vi "rszvl_core_global.vi"() -> ()   [LabVIEW 2014] (continued)
Callback"="", "Write Callback"="", "Range Callback"="", "Check Callback"="", "Rngtable Callback"="", "Coerce Callback"="", "User Callback"="", "Supported Models"="", "Instrument Options"="", "Repeated Capabilities"="", "Restricted Repeated Capabilities"="", "Help"="This attribute initiates an instrument reset.\n\nAvailable Repeated Capabilities:\nNone\n\nRemote-control command(s):\nSYSTem:PRESet", "Flags"={"OPC Wait"=FALSE, "Dont check status"=FALSE, "*WAI"=FALSE}, "Check Status Callback"=""}, {"Level"=2, "Descriptive Name"="System Version", "Class Only"=FALSE, "Data Type"=2, "Access"=0, "Identifier"="RSZVL_ATTR_SYST_VERSION", "Range Table"="", "Command"="SYST:VERS?", "Read Callback"="", "Write Callback"="", "Range Callback"="", "Check Callback"="", "Rngtable Callback"="", "Coerce Callback"="", "User Callback"="", "Supported Models"="", "Instrument Options"="", "Repeated Capabilities"="", "Restricted Repeated Capabilities"="", "Help"="This attribute queries the system version.\n\nAvailable Repeated Capabilities:\nNone\n\nRemote-control command(s):\nSYSTem:VERSion?", "Flags"={"OPC Wait"=FALSE, "Dont check status"=FALSE, "*WAI"=FALSE}, "Check Status Callback"=""}, {"Level"=2, "Descriptive Name"="Speaker Volume", "Class Only"=FALSE, "Data Type"=1, "Access"=2, "Identifier"="RSZVL_ATTR_SYST_SPEAKER", "Range Table"="rszvl_rngSpeakerVolume", "Command"="SYST:SPE:VOL", "Read Callback"="", "Write Callback"="", "Range Callback"="", "Check Callback"="", "Rngtable Callback"="", "Coerce Callback"="", "User Callback"="", "Supported Models"="", "Instrument Options"="", "Repeated Capabilities"="", "Restricted Repeated Capabilities"="", "Help"="This attribute sets the volume of the built-in loudspeaker for demodulated signals.\n\nAvailable Repeated Capabilities:\nNone\n\nRemote-control command(s):\nSYSTem:SPEaker:VOLume", "Flags"={"OPC Wait"=FALSE, "Dont check status"=FALSE, "*WAI"=FALSE}, "Check Status Callback"=""}, {"Level"=1, "Descriptive Name"="NWA Channel", "Class Only"=TRUE, "Data Type"=0, "Access"=0, "Identifier"="", "Range Table"="", "Command"="", "Read Callback"="", "Write Callback"="", "Range Callback"="", "Check Callback"="", "Rngtable Callback"="", "Coerce Callback"="", "User Callback"="", "Supported Models"="", "Instrument Options"="", "Repeated Capabilities"="", "Restricted Repeated Capabilities"="", "Help"="(1) NWA Number Of Sweeps:\nThis attribute defines the number of sweeps to be measured in single sweep mode (INITiate<Ch>:CONTinuous OFF). \n\n(2) NWA Averaging State:\nThis attribute enable or disable the sweep average.\n\n(3) NWA Averaging Count:\nThis attribute defines the number of consecutive sweeps to be combined for the sweep average (Average Factor).\n\n(4) NWA Restart Average:\nThis attribute starts a new average cycle, clearing all previous results and thus eliminating their effect on the new cycle. \n\n(5) NWA Resolution Bandwidth:\nThis attribute defines the resolution bandwidth of the analyzer (Meas Bandwidth).\n\n(6) NWA Sweep Points:\nThis attribute defines the total number of measurement points per sweep (Number of Points).\n\n(7) NWA Channel State:\nThis attribute creates or deletes channel no. <Ch> and selects it as the active channel. \n\n(8) NWA Channel Name:\nThis attribute assigns a name to channel number <Ch>. The channel must be created before (CONFigure:CHANnel<Ch>[:STATe] ON). Moreover it is not possible to assign the same name to two different channels.\n\n(9) NWA Assign Trace:\nThis attribute assigns an existing trace to a diagram area, using the <WndTr> suffix, and displays the trace.", "Flags"={"OPC Wait"=FALSE, "Dont check status"=FALSE, "*WAI"=FALSE}, "Check Status Callback"=""}, {"Level"=2, "Descriptive Name"="NWA Number Of Sweeps", "Class Only"=FALSE, "Data Type"=0, "Access"=2, "Identifier"="RSZVL_ATTR_NWA_NUMBER_OF_SWEEPS", "Range Table"="rszvl_rngNWANumberOfSweeps", "Command"="SENS:SWE:COUN", "Read Callback"="", "Write Callback"="", "Range Callback"="", "Check Callback"="", "Rngtable Callback"="", "Coerce Callback"="", "User Callback"="", "Supported Models"="", "Instrument Options"="", "Repeated Capabilities"="", "Restricted Repeated Capabilities"="", "Help"="This attribute defines the number of sweeps to be measured in single sweep mode (INITiate<Ch>:CONTinuous OFF).\n\nAvailable Repeated Capabilities:\nNone\n\nRemote-control command(s):\n[SENSe<1|2>:]SWEep:COUNt", "Flags"={"OPC Wait"=FALSE, "Dont check status"=FALSE, "*WAI"=FALSE}, "Check Status Callback"=""}, {"Level"=2, "Descriptive Name"="NWA Averaging State", "Class Only"=FALSE, "Data Type"=3, "Access"=2, "Identifier"="RSZVL_ATTR_NWA_AVG_STATE", "Range Table"="", "Command"="SENS{Channel}:AVER:STAT", "Read Callback"="", "Write Callback"="", "Range Callback"="", "Check Callback"="", "Rngtable Callback"="", "Coerce Callback"="", "User Callback"="", "Supported Models"="", "Instrument Options"="", "Repeated Capabilities"="", "Restricted Repeated Capabilities"="", "Help"="This attribute enable or disable the sweep average.\n\nAvailable Repeated Capabilities:\nChannel: CH1,CH2,CH3,CH4,CH5,CH6,CH7,CH8,CH9,CH10,CH11,CH12,CH13,CH14,CH15,CH16,CH17,CH18,CH19,CH20\r\n\nRemote-control command(s):\n[SENSe<Ch>:]AVERage[:STATe] ON | OFF", "Flags"={"OPC Wait"=FALSE, "Dont check status"=FALSE, "*WAI"=FALSE}, "Check Status Callback"=""}, {"Level"=2, "Descriptive Name"="NWA Averaging Count", "Class Only"=FALSE, "Data Type"=0, "Access"=2, "Identifier"="RSZVL_ATTR_NWA_AVG_COUNT", "Range Table"="rszvl_rngNWAAvgCount", "Command"="SENS{Channel}:AVER:COUN", "Read Callback"="", "Write Callback"="", "Range Callback"="", "Check Callback"="", "Rngtable Callback"="", "Coerce Callback"="", "User Callback"="", "Supported Models"="", "Instrument Options"="", "Repeated Capabilities"="", "Restricted Repeated Capabilities"="", "Help"="This attribute defines the number of consecutive sweeps to be combined for the sweep average (Average Factor).\n\nAvailable Repeated Capabilities:\nChannel: CH1,CH2,CH3,CH4,CH5,CH6,CH7,CH8,CH9,CH10,CH11,CH12,CH13,CH14,CH15,CH16,CH17,CH18,CH19,CH20\r\n\nRemote-control command(s):\n[SENSe<Ch>:]AVERage:COUNt", "Flags"={"OPC Wait"=FALSE, "Dont check status"=FALSE, "*WAI"=FALSE}, "Check Status Callback"=""}, {"Level"=2, "Descriptive Name"="NWA Restart Average", "Class Only"=FALSE, "Data Type"=4, "Access"=1, "Identifier"="RSZVL_ATTR_NWA_AVERAGE_CLEAR", "Range Table"="", "Command"="SENS{Channel}:AVER:CLE", "Read Callback"="", "Write Callback"="", "Range Callback"="", "Check Callback"="", "Rngtable Callback"="", "Coerce Callback"="", "User Callback"="", "Supported Models"="", "Instrument Options"="", "Repeated Capabilities"="", "Restricted Repeated Capabilities"="", "Help"="This attribute starts a new average cycle, clearing all previous results and thus eliminating their effect on the new cycle.\n\nAvailable Repeated Capabilities:\nChannel: CH1,CH2,CH3,CH4,CH5,CH6,CH7,CH8,CH9,CH10,CH11,CH12,CH13,CH14,CH15,CH16,CH17,CH18,CH19,CH20\r\n\nRemote-control command(s):\n[SENSe<Ch>:]AVERage:CLEar", "Flags"={"OPC Wait"=FALSE, "Dont check status"=FALSE, "*WAI"=FALSE}, "Check Status Callback"=""}, {"Level"=2, "Descriptive Name"="NWA Resolution Bandwidth", "Class Only"=FALSE, "Data Type"=1, "Access"=2, "Identifier"="RSZVL_ATTR_NWA_RESOLUTION_BANDWIDTH", "Range Table"="rszvl_rngNWARBW", "Command"="SENS{Channel}:BAND", "Read Callback"="", "Write Callback"="", "Range Callback"="", "Check Callback"="", "Rngtable Callback"="", "Coerce Callback"="", "User Callback"="", "Supported Models"="", "Instrument Options"="", "Repeated Capabilities"="", "Restricted Repeated Capabilities"="", "Help"="This attribute defines the resolution bandwidth of the analyzer (Meas Bandwidth).\n\nAvailable Repeated Capabilities:\nChannel: CH1,CH2,CH3,CH4,CH5,CH6,CH7,CH8,CH9,CH10,CH11,CH12,CH13,CH14,CH15,CH16,CH17,CH18,CH19,CH20\r\n\nRemote-control command(s):\n[SENSe<Ch>:]BANDwidth|BWIDth[:RESolution]", "Flags"={"OPC Wait"=FALSE, "Dont check status"=FALSE, "*WAI"=FALSE}, "Check Status Callback"=""}, {"Level"=2, "Descriptive Name"="NWA Sweep Points", "Class Only"=FALSE, "Data Type"=0, "Access"=2, "Identifier"="RSZVL_ATTR_NWA_SWEEP_POINTS", "Range Table"="rszvl_rngNWASwePoints", "Command"="SENS{Channel}:SWE:POIN", "Read Callback"="", "Write Callback"="", "Range Callback"="", "Check Callback"="", "Rngtable Callback"="", "Coerce Callback"="", "User Callback"="", "Supported Models"="", "Instrument Options"="", "Repeated Capabilities"="", "Restricted Repeated Capabilities"="", "Help"="This attribute defines the total number of measurement points per sweep (Number of Points).\n\nAvailable Repeated Capabilities:\nChannel: CH1,CH2,CH3,CH4,CH5,CH6,CH7,CH8,CH9,CH10,CH11,CH12,CH13,CH14,CH15,CH16,CH17,CH18,CH19,CH20\r\n\nRemote-control command(s):\n[SENSe<Ch>:]SWEep:POINts", "Flags"={"OPC Wait"=FALSE, "Dont check status"=FALSE, "*WAI"=FALSE}, "Check Status Callback"=""}, {"Level"=2, "Descriptive Name"="NWA Channel State", "Class Only"=FALSE, "Data Type"=3, "Access"=2, "Identifier"="RSZVL_ATTR_NWA_CHANNEL_STATE", "Range Table"="", "Command"="CONF:CHAN{Channel}:STAT", "Read Callback"="", "Write Callback"="", "Range Callback"="", "Check Callback"="", "Rngtable Callback"="", "Coerce Callback"="", "User Callback"="", "Supported Models"="", "Instrument Options"="", "Repeated Capabilities"="", "Restricted Repeated Capabilities"="", "Help"="This attribute creates or deletes channel no. <Ch> and selects it as the active channel.\n\nAvailable Repeated Capabilities:\nChannel: CH1,CH2,CH3,CH4,CH5,CH6,CH7,CH8,CH9,CH10,CH11,CH12,CH13,CH14,CH15,CH16,CH17,CH18,CH19,CH20\r\n\nRemote-control command(s):\nCONFigure:CHANnel<Ch>[:STATe] ON | OFF", "Flags"={"OPC Wait"=FALSE, "Dont check status"=FALSE, "*WAI"=FALSE}, "Check Status Callback"=""}, {"Level"=2, "Descriptive Name"="NWA Channel Name", "Class Only"=FALSE, "Data Type"=2, "Access"=2, "Identifier"="RSZVL_ATTR_NWA_CHANNEL_NAME", "Range Table"="", "Command"="CONF:CHAN{Channel}:NAME", "Read Callback"="rszvl_quotedString_ReadCallback.vi", "Write Callback"="rszvl_quotedString_WriteCallback.vi", "Range Callback"="", "Check Callback"="", "Rngtable Callback"="", "Coerce Callback"="", "User Callback"="", "Supported Models"="", "Instrument Options"="", "Repeated Capabilities"="", "Restricted Repeated Capabilities"="", "Help"="This attribute assigns a name to channel number <Ch>. The channel must be created before (CONFigure:CHANnel<Ch>[:STATe] ON). Moreover it is not possible to assign the same name to two different channels.\n\nAvailable Repeated Capabilities:\nChannel: CH1,CH2,CH3,CH4,CH5,CH6,CH7,CH8,CH9,CH10,CH11,CH12,CH13,CH14,CH15,CH16,CH17,CH18,CH19,CH20\r\n\nRemote-control command(s):\nCONFigure:CHANnel<Ch>:NAME '<Ch_name>'", "Flags"={"OPC Wait"=FALSE, "Dont check status"=FALSE, "*WAI"=FALSE}, "Check Status Callback"=""}, {"Level"=2, "Descriptive Name"="NWA Assign Trace", "Class Only"=FALSE, "Data Type"=2, "Access"=2, "Identifier"="RSZVL_ATTR_NWA_ASSIGN_TRACE", "Range Table"="", "Command"="DISP:WIND{DiagramArea}:TRAC{Trace}:FEED", "Read Callback"="rszvl_quotedString_ReadCallback.vi", "Write Callback"="rszvl_quotedString_WriteCallback.vi", "Range Callback"="", "Check Callback"="", "Rngtable Callback"="", "Coerce Callback"="", "User Callback"="", "Supported Models"="", "Instrument Options"="", "Repeated Capabilities"="", "Restricted Repeated Capabilities"="", "Help"="This attribute assigns an existing trace to a diagram area, using the <WndTr> suffix, and displays the trace.\n\nAvailable Repeated Capabilities:\nDiagramArea: DA1,DA2,DA3,DA4,DA5,DA6,DA7,DA8,DA9,DA10\r\nTrace: TR1,TR2,TR3,TR4,TR5,TR6,TR7,TR8,TR9,TR10,TR11,TR12,TR13,TR14,TR15,TR16,TR17,TR18,TR19,TR20\r\n\nRemote-control command(s):\nDISPlay[:WINDow<Wnd>]:TRACe<WndTr>:FEED '<trace_name>'", "Flags"={"OPC Wait"=FALSE, "Dont check status"=FALSE, "*WAI"=FALSE}, "Check Status Callback"=""}, {"Level"=1, "Descriptive Name"="NWA Stimulus", "Class Only"=TRUE, "Data Type"=0, "Access"=0, "Identifier"="", "Range Table"="", "Command"="", "Read Callback"="", "Write Callback"="", "Range Callback"="", "Check Callback"="", "Rngtable Callback"="", "Coerce Callback"="", "User Callback"="", "Supported Models"="", "Instrument Options"="", "Repeated Capabilities"="", "Restricted Repeated Capabilities"="", "Help"="(1) NWA Source Port:\nThis attribute selects a source port for the stimulus signal (Drive Port). The setting acts on the active trace.", "Flags"={"OPC Wait"=FALSE, "Dont check status"=FALSE, "*WAI"=FALSE}, "Check Status Callback"=""}, {"Level"=2, "Descriptive Name"="NWA Source Port", "Class Only"=FALSE, "Data Type"=0, "Access"=2, "Identifier"="RSZVL_ATTR_NWA_SOURCE_PORT", "Range Table"="rszvl_rngNWASourcePort", "Command"="SENS{Channel}:SWE:SRCP", "Read Callback"="", "Write Callback"="", "Range Callback"="", "Check Callback"="", "Rngtable Callback"="", "Coerce Callback"="", "User Callback"="", "Supported Models"="", "Instrument Options"="", "Repeated Capabilities"="", "Restricted Repeated Capabilities"="", "Help"="This attribute selects a source port for the stimulus signal (Drive Port). The setting acts on the active trace.\n\nAvailable Repeated Capabilities:\nChannel: CH1,CH2,CH3,CH4,CH5,CH6,CH7,CH8,CH9,CH10,CH11,CH12,CH13,CH14,CH15,CH16,CH17,CH18,CH19,CH20\r\n\nRemote-control command(s):\n[SENSe<Chn>:]SWEep:SRCPort 1 | 2", "Flags"={"OPC Wait"=FALSE, "Dont check status"=FALSE, "*WAI"=FALSE}, "Check Status Callback"=""}, {"Level"=2, "Descriptive Name"="NWA RF Output", "Class Only"=FALSE, "Data Type"=3, "Access"=2, "Identifier"="RSZVL_ATTR_NWA_RF_OUTPUT", "Range Table"="", "Command"="OUTP:STAT", "Read Callback"="", "Write Callback"="", "Range Callback"="", "Check Callback"="", "Rngtable Callback"="", "Coerce Callback"="", "User Callback"="", "Supported Models"="", "Instrument Options"="", "Repeated Capabilities"="", "Restricted Repeated Capabilities"="", "Help"="This attribute turns the internal source power at all ports and the power of all external generators on or off.\n\nAvailable Repeated Capabilities:\nNone\n\nRemote-control command(s):\nOUTPut<Ch>[:STATe] ON | OFF", "Flags"={"OPC Wait"=FALSE, "Dont check status"=FALSE, "*WAI"=FALSE}, "Check Status Callback"=""}, {"Level"=1, "Descriptive Name"="NWA Sweep", "Class Only"=TRUE, "Data Type"=0, "Access"=0, "Identifier"="", "Range Table"="", "Command"="", "Read Callback"="", "Write Callback"="", "Range Callback"="", "Check Callback"="", "Rngtable Callback"="", "Coerce Callback"="", "User Callback"="", "Supported Models"="", "Instrument Options"="", "Repeated Capabilities"="", "Restricted Repeated Capabilities"="", "Help"="(1) NWA Sweep Type:\nThis attribute selects the sweep type (frequency) and the position of the sweep points across the sweep range. \n\n(2) NWA Sweep Meas Delay:\nThis attribute defines the Meas. Delay time for each partial measurement.\n\n(3) NWA Sweep Step:\nThis attribute sets the distance between two consecutive sweep points.\n\n(4) NWA Sweep Segment (Class):\nPut a help here", "Flags"={"OPC Wait"=FALSE, "Dont check status"=FALSE, "*WAI"=FALSE}, "Check Status Callback"=""}, {"Level"=2, "Descriptive Name"="NWA Sweep Type", "Class Only"=FALSE, "Data Type"=0, "Access"=2, "Identifier"="RSZVL_ATTR_NWA_SWEEP_TYPE", "Range Table"="rszvl_rngNWASweepType", "Command"="SENS{Channel}:SWE:TYPE", "Read Callback"="", "Write Callback"="", "Range Callback"="", "Check Callback"="", "Rngtable Callback"="", "Coerce Callback"="", "User Callback"="", "Supported Models"="", "Instrument Options"="", "Repeated Capabilities"="", "Restricted Repeated Capabilities"="", "Help"="This attribute selects the sweep type (frequency) and the position of the sweep points across the sweep range.\n\nAvailable Repeated Capabilities:\nChannel: CH1,CH2,CH3,CH4,CH5,CH6,CH7,CH8,CH9,CH10,CH11,CH12,CH13,CH14,CH15,CH16,CH17,CH18,CH19,CH20\r\n\nRemote-control command(s):\n[SENSe<Ch>:]SWEep:TYPE LINear | LOGarithmic | SEGMent", "Flags"={"OPC Wait"=FALSE, "Dont check status"=FALSE, "*WAI"=FALSE}, "Check Status Callback"=""}, {"Level"=2, "Descriptive Name"="NWA Sweep Meas Delay", "Class Only"=FALSE, "Data Type"=1, "Access"=2, "Identifier"="RSZVL_ATTR_NWA_SWEEP_MEAS_DELAY", "Range Table"="rszvl_rngNWASweepMeasDelay", "Command"="SENS{Channel}:SWE:DWEL", "Read Callback"="", "Write Callback"="", "Range Callback"="", "Check Callback"="", "Rngtable Callback"="", "Coerce Callback"="", "User Callback"="", "Supported Models"="", "Instrument Options"="", "Repeated Capabilities"="", "Restricted Repeated Capabilities"="", "Help"="This attribute defines the Meas. Delay time for each partial measurement. Not available for ZVL13.\n\nAvailable Repeated Capabilities:\nChannel: CH1,CH2,CH3,CH4,CH5,CH6,CH7,CH8,CH9,CH10,CH11,CH12,CH13,CH14,CH15,CH16,CH17,CH18,CH19,CH20\r\n\nRemote-control command(s):\n[SENSe<Ch>:]SWEep:DWELl", "Flags"={"OPC Wait"=FALSE, "Dont check status"=FALSE, "*WAI"=FALSE}, "Check Status Callback"=""}, {"Level"=2, "Descriptive Name"="NWA Sweep Step", "Class Only"=FALSE, "Data Type"=1, "Access"=2, "Identifier"="RSZVL_ATTR_NWA_SWEEP_STEP", "Range Table"="", "Command"="SENS{Channel}:SWE:STEP", "Read Callback"="", "Write Callback"="", "Range Callback"="", "Check Callback"="", "Rngtable Callback"="", "Coerce Callback"="", "User Callback"="", "Supported Models"="", "Instrument Options"="", "Repeated Capabilities"="", "Restricted Repeated Capabilities"="", "Help"="This attribute sets the distance between two consecutive sweep points.\n\nAvailable Repeated Capabilities:\nChannel: CH1,CH2,CH3,CH4,CH5,CH6,CH7,CH8,CH9,CH10,CH11,CH12,CH13,CH14,CH15,CH16,CH17,CH18,CH19,CH20\r\n\nRemote-control command(s):\n[SENSe<Ch>:]SWEep:STEP", "Flags"={"OPC Wait"=FALSE, "Dont check status"=FALSE, "*WAI"=FALSE}, "Check Status Callback"=""}, {"Level"=2, "Descriptive Name"="NWA Sweep Segment", "Class Only"=TRUE, "Data Type"=0, "Access"=0, "Identifier"="", "Range Table"="", "Command"="", "Read Callback"="", "Write Callback"="", "Range Callback"="", "Check Callback"="", "Rngtable Callback"="", "Coerce Callback"="", "User Callback"="", "Supported Models"="", "Instrument Options"="", "Repeated Capabilities"="", "Restricted Repeated Capabilities"="", "Help"="Put a help here", "Flags"={"OPC Wait"=FALSE, "Dont check status"=FALSE, "*WAI"=FALSE}, "Check Status Callback"=""}, {"Level"=3, "Descriptive Name"="NWA Insert New Segment", "Class Only"=FALSE, "Data Type"=4, "Access"=1, "Identifier"="RSZVL_ATTR_NWA_INSERT_NEW_SEGMENT", "Range Table"="", "Command"="SENS{Channel}:SEGM{Segment}:ADD", "Read Callback"="", "Write Callback"="", "Range Callback"="", "Check Callback"="", "Rngtable Callback"="", "Coerce Callback"="", "User Callback"="", "Supported Models"="", "Instrument Options"="", "Repeated Capabilities"="", "Restricted Repeated Capabilities"="", "Help"="This attribute inserts a new sweep segment using default channel settings. The added segment covers the frequency interval between the maximum frequency of the existing sweep segments and the stop frequency of the entire sweep range.\n\nAvailable Repeated Capabilities:\nChannel: CH1,CH2,CH3,CH4,CH5,CH6,CH7,CH8,CH9,CH10,CH11,CH12,CH13,CH14,CH15,CH16,CH17,CH18,CH19,CH20\r\nSegment: SEG1,SEG2,SEG3,SEG4,SEG5,SEG6,SEG7,SEG8,SEG9,SEG10,SEG11,SEG12,SEG13,SEG14,SEG15,SEG16,SEG17,SEG18,SEG19,SEG20\r\n\nRemote-control command(s):\n[SENSe<Ch>:]SEGMent<Seg>:ADD", "Flags"={"OPC Wait"=FALSE, "Dont check status"=FALSE, "*WAI"=FALSE}, "Check Status Callback"=""}, {"Level"=3, "Descriptive Name"="NWA Segment Select Sweep Time", "Class Only"=FALSE, "Data Type"=0, "Access"=2, "Identifier"="RSZVL_ATTR_NWA_SEGMENT_SELECT_SWEEP_TIME", "Range Table"="rszvl_rngNWASegmentSelectSweepTime", "Command"="SENS{Channel}:SEGM{Segment}:INS:SEL", "Read Callback"="", "Write Callback"="", "Range Callback"="", "Check Callback"="", "Rngtable Callback"="", "Coerce Callback"="", "User Callback"="", "Supported Models"="", "Instrument Options"="", "Repeated Capabilities"="", "Restricted Repeated Capabilities"="", "Help"="This attribute defines whether the sweep time of a new segment is entered as a segment sweep time or as a meas. delay.\n\nAvailable Repeated Capabilities:\nChannel: CH1,CH2,CH3,CH4,CH5,CH6,CH7,CH8,CH9,CH10,CH11,CH12,CH13,CH14,CH15,CH16,CH17,CH18,CH19,CH20\r\nSegment: SEG1,SEG2,SEG3,SEG4,SEG5,SEG6,SEG7,SEG8,SEG9,SEG10,SEG11,SEG12,SEG13,SEG14,SEG15,SEG16,SEG17,SEG18,SEG19,SEG20\r\n\nRemote-control command(s):\n[SENSe<Ch>:]SEGMent<Seg>:INSert:SELect SWTime | DWELl", "Flags"={"OPC Wait"=FALSE, "Dont check status"=FALSE, "*WAI"=FALSE}, "Check Status Callback"=""}, {"Level"=3, "Descriptive Name"="NWA Segment State", "Class Only"=FALSE, "Data Type"=3, "Access"=2, "Identifier"="RSZVL_ATTR_NWA_SEGMENT_STATE", "Range Table"="", "Command"="SENS{Channel}:SEGM{Segment}:STAT", "Read Callback"="", "Write Callback"="", "Range Callback"="", "Check Callback"="", "Rngtable Callback"="", "Coerce Callback"="", "User Callback"="", "Supported Models"="", "Instrument Options"="", "Repeated Capabilities"="", "Restricted Repeated Capabilities"="", "Help"="This attribute activates or deactivates the sweep segment <Seg>. Sweep points belonging to inactive segments only are not measured.\n\nAvailable Repeated Capabilities:\nChannel: CH1,CH2,CH3,CH4,CH5,CH6,CH7,CH8,CH9,CH10,CH11,CH12,CH13,CH14,CH15,CH16,CH17,CH18,CH19,CH20\r\nSegment: SEG1,SEG2,SEG3,SEG4,SEG5,SEG6,SEG7,SEG8,SEG9,SEG10,SEG11,SEG12,SEG13,SEG14,SEG15,SEG16,SEG17,SEG18,SEG19,SEG20\r\n\nRemote-control command(s):\n[SENSe<Ch>:]SEGMent<Seg>[:STATe] ON | OFF", "Flags"={"OPC Wait"=FALSE, "Dont check status"=FALSE, "*WAI"=FALSE}, "Check Status Callback"=""}, {"Level"=3, "Descriptive Name"="NWA Segment Frequency Start", "Class Only"=FALSE, "Data Type"=1, "Access"=2, "Identifier"="RSZVL_ATTR_NWA_SEGMENT_FREQ_START", "Range Table"="", "Command"="SENS{Channel}:SEGM{Segment}:FREQ:STAR", "Read Callback"="", "Write Callback"="", "Range Callback"="", "Check Callback"="", "Rngtable Callback"="", "Coerce Callback"="", "User Callback"="", "Supported Models"="", "Instrument Options"="", "Repeated Capabilities"="", "Restricted Repeated Capabilities"="", "Help"="This attribute defines the Start frequency of sweep segment no. <Seg>.\n\nAvailable Repeated Capabilities:\nChannel: CH1,CH2,CH3,CH4,CH5,CH6,CH7,CH8,CH9,CH10,CH11,CH12,CH13,CH14,CH15,CH16,CH17,CH18,CH19,CH20\r\nSegment: SEG1,SEG2,SEG3,SEG4,SEG5,SEG6,SEG7,SEG8,SEG9,SEG10,SEG11,SEG12,SEG13,SEG14,SEG15,SEG16,SEG17,SEG18,SEG19,SEG20\r\n\nRemote-control command(s):\n[SENSe<Ch>:]SEGMent<Seg>:FREQuency:STARt", "Flags"={"OPC Wait"=FALSE, "Dont check status"=FALSE, "*WAI"=FALSE}, "Check Status Callback"=""}, {"Level"=3, "Descriptive Name"="NWA Segment Frequency Stop", "Class Only"=FALSE, "Data Type"=1, "Access"=2, "Identifier"="RSZVL_ATTR_NWA_SEGMENT_FREQ_STOP", "Range Table"="", "Command"="SENS{Channel}:SEGM{Segment}:FREQ:STOP", "Read Callback"="", "Write Callback"="", "Range Callback"="", "Check Callback"="", "Rngtable Callback"="", "Coerce Callback"="", "User Callback"="", "Supported Models"="", "Instrument Options"="", "Repeated Capabilities"="", "Restricted Repeated Capabilities"="", "Help"="This attribute defines the Stop frequency of sweep segment no. <Seg>.\n\nAvailable Repeated Capabilities:\nChannel: CH1,CH2,CH3,CH4,CH5,CH6,CH7,CH8,CH9,CH10,CH11,CH12,CH13,CH14,CH15,CH16,CH17,CH18,CH19,CH20\r\nSegment: SEG1,SEG2,SEG3,SEG4,SEG5,SEG6,SEG7,SEG8,SEG9,SEG10,SEG11,SEG12,SEG13,SEG14,SEG15,SEG16,SEG17,SEG18,SEG19,SEG20\r\n\nRemote-control command(s):\n[SENSe<Ch>:]SEGMent<Seg>:FREQuency:STOP", "Flags"={"OPC Wait"=FALSE, "Dont check status"=FALSE, "*WAI"=FALSE}, "Check Status Callback"=""}, {"Level"=3, "Descriptive Name"="NWA Segment Power Control", "Class Only"=FALSE, "Data Type"=3, "Access"=2, "Identifier"="RSZVL_ATTR_NWA_SEGMENT_POWER_CONTROL", "Range Table"="", "Command"="SENS{Channel}:SEGM{Segment}:POW:LEV:CONT", "Read Callback"="", "Write Callback"="", "Range Callback"="", "Check Callback"="", "Rngtable Callback"="", "Coerce Callback"="", "User Callback"="", "Supported Models"="", "Instrument Options"="", "Repeated Capabilities"="", "Restricted Repeated Capabilities"="", "Help"="This attribute qualifies whether or not the Power of the internal signal source can be set independently for each sweep segment.\n\nAvailable Repeated Capabilities:\nChannel: CH1,CH2,CH3,CH4,CH5,CH6,CH7,CH8,CH9,CH10,CH11,CH12,CH13,CH14,CH15,CH16,CH17,CH18,CH19,CH20\r\nSegment: SEG1,SEG2,SEG3,SEG4,SEG5,SEG6,SEG7,SEG8,SEG9,SEG10,SEG11,SEG12,SEG13,SEG14,SEG15,SEG16,SEG17,SEG18,SEG19,SEG20\r\n\nRemote-control command(s):\n[SENSe<Ch>:]SEGMent<Seg>:POWer[:LEVel]:CONTrol ON | OFF", "Flags"={"OPC Wait"=FALSE, "Dont check status"=FALSE, "*WAI"=FALSE}, "Check Status Callback"=""}, {"Level"=3, "Descriptive Name"="NWA Segment Attenuation", "Class Only"=FALSE, "Data Type"=1, "Access"=2, "Identifier"="RSZVL_ATTR_NWA_SEGMENT_ATTEN", "Range Table"="rszvl_rngNWASegmentAtten", "Command"="SENS{Channel}:SEGM{Segment}:ATT{Port}", "Read Callback"="", "Write Callback"="", "Range Callback"="", "Check Callback"="", "Rngtable Callback"="", "Coerce Callback"="", "User Callback"="", "Supported Models"="", "Instrument Options"="", "Repeated Capabilities"="", "Restricted Repeated Capabilities"="", "Help"="This attribute defines the attenuation factors for the received waves b1 and b2 in segment no. <Seg>.\n\nAvailable Repeated Capabilities:\nChannel: CH1,CH2,CH3,CH4,CH5,CH6,CH7,CH8,CH9,CH10,CH11,CH12,CH13,CH14,CH15,CH16,CH17,CH18,CH19,CH20\r\nSegment: SEG1,SEG2,SEG3,SEG4,SEG5,SEG6,SEG7,SEG8,SEG9,SEG10,SEG11,SEG12,SEG13,SEG14,SEG15,SEG16,SEG17,SEG18,SEG19,SEG20\r\nPort: P1,P2,P3,P4,P5,P6,P7,P8,P9,P10\r\n\nRemote-control command(s):\n[SENSe<Ch>:]SEGMent<Seg>:ATTenuation<port_no> <Attenuation>", "Flags"={"OPC Wait"=FALSE, "Dont check status"=FALSE, "*WAI"=FALSE}, "Check Status Callback"=""}, {"Level"=3, "Descriptive Name"="NWA Segment Bandwidth Control", "Class Only"=FALSE, "Data Type"=3, "Access"=2, "Identifier"="RSZVL_ATTR_NWA_SEGMENT_BAND_CONTROL", "Range Table"="", "Command"="SENS{Channel}:SEGM{Segment}:BWID:RES:CONT", "Read Callback"="", "Write Callback"="", "Range Callback"="", "Check Callback"="", "Rngtable Callback"="", "Coerce Callback"="", "User Callback"="", "Supported Models"="", "Instrument Options"="", "Repeated Capabilities"="", "Restricted Repeated Capabilities"="", "Help"="This attribute qualifies whether or not the Meas Bandwidth can be set independently for each sweep segment.\n\nAvailable Repeated Capabilities:\nChannel: CH1,CH2,CH3,CH4,CH5,CH6,CH7,CH8,CH9,CH10,CH11,CH12,CH13,CH14,CH15,CH16,CH17,CH18,CH19,CH20\r\nSegment: SEG1,SEG2,SEG3,SEG4,SEG5,SEG6,SEG7,SEG8,SEG9,SEG10,SEG11,SEG12,SEG13,SEG14,SEG15,SEG16,SEG17,SEG18,SEG19,SEG20\r\n\nRemote-control command(s):\n[SENSe<Ch>:]SEGMent<Seg>:BWIDth[:RESolution]:CONTrol ON | OFF", "Flags"={"OPC Wait"=FALSE, "Dont check status"=FALSE, "*WAI"=FALSE}, "Check Status Callback"=""}, {"Level"=3, "Descriptive Name"="NWA Segment Selectivity Control", "Class Only"=FALSE, "Data Type"=3, "Access"=2, "Identifier"="RSZVL_ATTR_NWA_SEGMENT_SELECT_CONTROL", "Range Table"="", "Command"="SENS{Channel}:SEGM{Segment}:BWID:RES:SEL:CONT", "Read Callback"="", "Write Callback"="", "Range Callback"="", "Check Callback"="", "Rngtable Callback"="", "Coerce Callback"="", "User Callback"="", "Supported Models"="", "Instrument Options"="", "Repeated Capabilities"="", "Restricted Repeated Capabilities"="", "Help"="This attribute qualifies whether or not the Filter Type (selectivity) can be set independently for each sweep segment.\n\nAvailable Repeated Capabilities:\nChannel: CH1,CH2,CH3,CH4,CH5,CH6,CH7,CH8,CH9,CH10,CH11,CH12,CH13,CH14,CH15,CH16,CH17,CH18,CH19,CH20\r\nSegment: SEG1,SEG2,SEG3,SEG4,SEG5,SEG6,SEG7,SEG8,SEG9,SEG10,SEG11,SEG12,SEG13,SEG14,SEG15,SEG16,SEG17,SEG18,SEG19,SEG20\r\n\nRemote-control command(s):\n[SENSe<Ch>:]SEGMent<Seg>:BWIDth[:RESolution]:SELect:CONTrol ON | OFF", "Flags"={"OPC Wait"=FALSE, "Dont check status"=FALSE, "*WAI"=FALSE}, "Check Status Callback"=""}, {"Level"=3, "Descriptive Name"="NWA Segment Time Control", "Class Only"=FALSE, "Data Type"=3, "Access"=2, "Identifier"="RSZVL_ATTR_NWA_SEGMENT_TIME_CONTROL", "Range Table"="", "Command"="SENS{Channel}:SEGM{Segment}:SWE:TIME:CONT", "Read Callback"="", "Write Callback"="", "Range Callback"="", "Check Callback"="", "Rngtable Callback"="", "Coerce Callback"="", "User Callback"="", "Supported Models"="", "Instrument Options"="", "Repeated Capabilities"="", "Restricted Repeated Capabilities"="", "Help"="This attribute qualifies whether or not the Segment Sweep Time can be set independently for each sweep segment.\n\nAvailable Repeated Capabilities:\nChannel: CH1,CH2,CH3,CH4,CH5,CH6,CH7,CH8,CH9,CH10,CH11,CH12,CH13,CH14,CH15,CH16,CH17,CH18,CH19,CH20\r\nSegment: SEG1,SEG2,SEG3,SEG4,SEG5,SEG6,SEG7,SEG8,SEG9,SEG10,SEG11,SEG12,SEG13,SEG14,SEG15,SEG16,SEG17,SEG18,SEG19,SEG20\r\n\nRemote-control command(s):\n[SENSe<Ch>:]SEGMent<Seg>:SWEep:TIME:CONTrol ON | OFF", "Flags"={"OPC Wait"=FALSE, "Dont check status"=FALSE, "*WAI"=FALSE}, "Check Status Callback"=""}, {"Level"=3, "Descriptive Name"="NWA Segment Meas Delay Control", "Class Only"=FALSE, "Data Type"=3, "Access"=2, "Identifier"="RSZVL_ATTR_NWA_SEGMENT_MEAS_DELAY_CONTROL", "Range Table"="", "Command"="SENS{Channel}:SEGM{Segment}:SWE:DWEL:CONT", "Read Callback"="", "Write Callback"="", "Range Callback"="", "Check Callback"="", "Rngtable Callback"="", "Coerce Callback"="", "User Callback"="", "Supported Models"="", "Instrument Options"="", "Repeated Capabilities"="", "Restricted Repeated Capabilities"="", "Help"="This attribute qualifies whether or not the Meas. Delay can be set independently for each sweep segment. Not available for ZVL13.\n\nAvailable Repeated Capabilities:\nChannel: CH1,CH2,CH3,CH4,CH5,CH6,CH7,CH8,CH9,CH10,CH11,CH12,CH13,CH14,CH15,CH16,CH17,CH18,CH19,CH20\r\nSegment: SEG1,SEG2,SEG3,SEG4,SEG5,SEG6,SEG7,SEG8,SEG9,SEG10,SEG11,SEG12,SEG13,SEG14,SEG15,SEG16,SEG17,SEG18,SEG19,SEG20\r\n\nRemote-control command(s):\n[SENSe<Ch>:]SEGMent<Seg>:SWEep:DWELl:CONTrol ON | OFF", "Flags"={"OPC Wait"=FALSE, "Dont check status"=FALSE, "*WAI"=FALSE}, "Check Status Callback"=""}, {"Level"=3, "Descriptive Name"="NWA Segment Resolution Bandwidth", "Class Only"=FALSE, "Data Type"=1, "Access"=2, "Identifier"="RSZVL_ATTR_NWA_SEGMENT_RES_BAND", "Range Table"="rszvl_rngNWASegmentRBW", "Command"="SENS{Channel}:SEGM{Segment}:BWID:RES", "Read Callback"="", "Write Callback"="", "Range Callback"="", "Check Callback"="", "Rngtable Callback"="", "Coerce Callback"="", "User Callback"="", "Supported Models"="", "Instrument Options"="", "Repeated Capabilities"="", "Restricted Repeated Capabilities"="", "Help"="This attribute defines the resolution bandwidth of the analyzer (Meas Bandwidth) in sweep segment no. <Seg>.\n\nAvailable Repeated Capabilities:\nChannel: CH1,CH2,CH3,CH4,CH5,CH6,CH7,CH8,CH9,CH10,CH11,CH12,CH13,CH14,CH15,CH16,CH17,CH18,CH19,CH20\r\nSegment: SEG1,SEG2,SEG3,SEG4,SEG5,SEG6,SEG7,SEG8,SEG9,SEG10,SEG11,SEG12,SEG13,SEG14,SEG15,SEG16,SEG17,SEG18,SEG19,SEG20\r\n\nRemote-control command(s):\n[SENSe<Ch>:]SEGMent<Seg>:BWIDth[:RESolution]", "Flags"={"OPC Wait"=FALSE, "Dont check status"=FALSE, "*WAI"=FALSE}, "Check Status Callback"=""}, {"Level"=3, "Descriptive Name"="NWA Segment Selectivity", "Class Only"=FALSE, "Data Type"=0, "Access"=2, "Identifier"="RSZVL_ATTR_NWA_SEGMENT_SELECTIVITY", "Range Table"="rszvl_rngNWASegmentSelectivity", "Command"="SENS{Channel}:SEGM{Segment}:BWID:RES:SEL", "Read Callback"="", "Write Callback"="", "Range Callback"="", "Check Callback"="", "Rngtable Callback"="", "Coerce Callback"="", "User Callback"="", "Supported Models"="", "Instrument Options"="", "Repeated Capabilities"="", "Restricted Repeated Capabilities"="", "Help"="This attribute defines the Filter Type (selectivity) in sweep segment no. <Seg>.\n\nAvailable Repeated Capabilities:\nChannel: CH1,CH2,CH3,CH4,CH5,CH6,CH7,CH8,CH9,CH10,CH11,CH12,CH13,CH14,CH15,CH16,CH17,CH18,CH19,CH20\r\nSegment: SEG1,SEG2,SEG3,SEG4,SEG5,SEG6,SEG7,SEG8,SEG9,SEG10,SEG11,SEG12,SEG13,SEG14,SEG15,SEG16,SEG17,SEG18,SEG19,SEG20\r\n\nRemote-control command(s):\n[SENSe<Ch>:]SEGMent<Seg>:BWIDth[:RESolution]:SELect FAST | NORMal", "Flags"={"OPC Wait"=FALSE, "Dont check status"=FALSE, "*WAI"=FALSE}, "Check Status Callback"=""}, {"Level"=3, "Descriptive Name"="NWA Segment Sweep Time", "Class Only"=FALSE, "Data Type"=1, "Access"=2, "Identifier"="RSZVL_ATTR_NWA_SEGMENT_SWEEP_TIME", "Range Table"="rszvl_rngNWASegmentSweepTime", "Command"="SENS{Channel}:SEGM{Segment}:SWE:TIME", "Read Callback"="", "Write Callback"="", "Range Callback"="", "Check Callback"="", "Rngtable Callback"="", "Coerce Callback"="", "User Callback"="", "Supported Models"="", "Instrument Options"="", "Repeated Capabilities"="", "Restricted Repeated Capabilities"="", "Help"="This attribute sets the duration of the sweep in sweep segment no. <Seg> (Segment Sweep Time).\n\nAvailable Repeated Capabilities:\nChannel: CH1,CH2,CH3,CH4,CH5,CH6,CH7,CH8,CH9,CH10,CH11,CH12,CH13,CH14,CH15,CH16,CH17,CH18,CH19,CH20\r\nSegment: SEG1,SEG2,SEG3,SEG4,SEG5,SEG6,SEG7,SEG8,SEG9,SEG10,SEG11,SEG12,SEG13,SEG14,SEG15,SEG16,SEG17,SEG18,SEG19,SEG20\r\n\nRemote-control command(s):\n[SENSe<Ch>:]SEGMent<Seg>:SWEep:TIME", "Flags"={"OPC Wait"=FALSE, "Dont check status"=FALSE, "*WAI"=FALSE}, "Check Status Callback"=""}, {"Level"=3, "Descriptive Name"="NWA Segment Meas Delay", "Class Only"=FALSE, "Data Type"=1, "Access"=2, "Identifier"="RSZVL_ATTR_NWA_SEGMENT_MEAS_DELAY", "Range Table"="rszvl_rngNWASegmentMeasDelay", "Command"="SENS{Channel}:SEGM{Segment}:SWE:DWEL", "Read Callback"="", "Write Callback"="", "Range Callback"="", "Check Callback"="", "Rngtable Callback"="", "Coerce Callback"="", "User Callback"="", "Supported Models"="", "Instrument Options"="", "Repeated Capabilities"="", "Restricted Repeated Capabilities"="", "Help"="This attribute defines the delay time for each partial measurement in sweep segment no. <Seg> (Meas. Delay). Not available for ZVL13.\n\nAvailable Repeated Capabilities:\nChannel: CH1,CH2,CH3,CH4,CH5,CH6,CH7,CH8,CH9,CH10,CH11,CH12,CH13,CH14,CH15,CH16,CH17,CH18,CH19,CH20\r\nSegment: SEG1,SEG2,SEG3,SEG4,SEG5,SEG6,SEG7,SEG8,SEG9,SEG10,SEG11,SEG12,SEG13,SEG14,SEG15,SEG16,SEG17,SEG18,SEG19,SEG20\r\n\nRemote-control command(s):\n[SENSe<Ch>:]SEGMent<Seg>:SWEep:DWELl", "Flags"={"OPC Wait"=FALSE, "Dont check status"=FALSE, "*WAI"=FALSE}, "Check Status Callback"=""}, {"Level"=3, "Descriptive Name"="NWA Segment Number Of Points", "Class Only"=FALSE, "Data Type"=0, "Access"=2, "Identifier"="RSZVL_ATTR_NWA_SEGMENT_SWEEP_POINTS", "Range Table"="rszvl_rngNWASegmentSweepPoints", "Command"="SENS{Channel}:SEGM{Segment}:SWE:POIN", "Read Callback"="", "Write Callback"="", "Range Callback"="", "Check Callback"="", "Rngtable Callback"="", "Coerce Callback"="", "User Callback"="", "Supported Models"="", "Instrument Options"="", "Repeated Capabilities"="", "Restricted Repeated Capabilities"="", "Help"="This attribute defines the total number of measurement Points in sweep segment no. <Seg>.\n\nAvailable Repeated Capabilities:\nChannel: CH1,CH2,CH3,CH4,CH5,CH6,CH7,CH8,CH9,CH10,CH11,CH12,CH13,CH14,CH15,CH16,CH17,CH18,CH19,CH20\r\nSegment: SEG1,SEG2,SEG3,SEG4,SEG5,SEG6,SEG7,SEG8,SEG9,SEG10,SEG11,SEG12,SEG13,SEG14,SEG15,SEG16,SEG17,SEG18,SEG19,SEG20\r\n\nRemote-control command(s):\n[SENSe<Ch>:]SEGMent<Seg>:SWEep:POINts", "Flags"={"OPC Wait"=FALSE, "Dont check status"=FALSE, "*WAI"=FALSE}, "Check Status Callback"=""}, {"Level"=3, "Descriptive Name"="NWA Segment Power", "Class Only"=FALSE, "Data Type"=1, "Access"=2, "Identifier"="RSZVL_ATTR_NWA_SEGMENT_POWER", "Range Table"="rszvl_rngNWASegmentPower", "Command"="SENS{Channel}:SEGM{Segment}:POW:LEV", "Read Callback"="", "Write Callback"="", "Range Callback"="", "Check Callback"="", "Rngtable Callback"="", "Coerce Callback"="", "User Callback"="", "Supported Models"="", "Instrument Options"="", "Repeated Capabilities"="", "Restricted Repeated Capabilities"="", "Help"="This attribute defines the Power of the internal signal source in sweep segment no. <Seg>. At the same time, the command activates separate power control in all sweep segments ([SENSe<Ch>:]SEGMent<Seg>:POWer[:Level]:CONTrol ON).\n\nAvailable Repeated Capabilities:\nChannel: CH1,CH2,CH3,CH4,CH5,CH6,CH7,CH8,CH9,CH10,CH11,CH12,CH13,CH14,CH15,CH16,CH17,CH18,CH19,CH20\r\nSegment: SEG1,SEG2,SEG3,SEG4,SEG5,SEG6,SEG7,SEG8,SEG9,SEG10,SEG11,SEG12,SEG13,SEG14,SEG15,SEG16,SEG17,SEG18,SEG19,SEG20\r\n\nRemote-control command(s):\n[SENSe<Ch>:]SEGMent<Seg>:POWer[:LEVel]", "Flags"={"OPC Wait"=FALSE, "Dont check status"=FALSE, "*WAI"=FALSE}, "Check Status Callback"=""}, {"Level"=3, "Descriptive Name"="NWA Segment Get Number Of Sweep Segments", "Class Only"=FALSE, "Data Type"=0, "Access"=0, "Identifier"="RSZVL_ATTR_NWA_SEGMENT_GET_COUNT", "Range Table"="", "Command"="SENS{Channel}:SEGM:COUN?", "Read Callback"="", "Write Callback"="", "Range Callback"="", "Check Callback"="", "Rngtable Callback"="", "Coerce Callback"="", "User Callback"="", "Supported Models"="", "Instrument Options"="", "Repeated Capabilities"="", "Restricted Repeated Capabilities"="", "Help"="This attribute returns the number of sweep segments in the channel including all segments that are switched off.\n\nAvailable Repeated Capabilities:\nChannel: CH1,CH2,CH3,CH4,CH5,CH6,CH7,CH8,CH9,CH10,CH11,CH12,CH13,CH14,CH15,CH16,CH17,CH18,CH19,CH20\r\n\nRemote-control command(s):\n[SENSe<Ch>:]SEGMent<Seg>:COUNt?", "Flags"={"OPC Wait"=FALSE, "Dont check status"=FALSE, "*WAI"=FALSE}, "Check Status Callback"=""}, {"Level"=3, "Descriptive Name"="NWA Segment Delete", "Class Only"=FALSE, "Data Type"=4, "Access"=1, "Identifier"="RSZVL_ATTR_NWA_SEGMENT_DELETE", "Range Table"="", "Command"="SENS{Channel}:SEGM{Segment}:DEL", "Read Callback"="", "Write Callback"="", "Range Callback"="", "Check Callback"="", "Rngtable Callback"="", "Coerce Callback"="", "User Callback"="", "Supported Models"="", "Instrument Options"="", "Repeated Capabilities"="", "Restricted Repeated Capabilities"="", "Help"="This attribute deletes the specified (single) sweep segment (Del. Selected Segment).\n\nAvailable Repeated Capabilities:\nChannel: CH1,CH2,CH3,CH4,CH5,CH6,CH7,CH8,CH9,CH10,CH11,CH12,CH13,CH14,CH15,CH16,CH17,CH18,CH19,CH20\r\nSegment: SEG1,SEG2,SEG3,SEG4,SEG5,SEG6,SEG7,SEG8,SEG9,SEG10,SEG11,SEG12,SEG13,SEG14,SEG15,SEG16,SEG17,SEG18,SEG19,SEG20\r\n\nRemote-control command(s):\n[SENSe<Ch>:]SEGMent<Seg>:DELete", "Flags"={"OPC Wait"=FALSE, "Dont check status"=FALSE, "*WAI"=FALSE}, "Check Status Callback"=""}, {"Level"=3, "Descriptive Name"="NWA Segment Delete All", "Class Only"=FALSE, "Data Type"=4, "Access"=1, "Identifier"="RSZVL_ATTR_NWA_SEGMENT_DELETE_ALL", "Range Table"="", "Command"="SENS{Channel}:SEGM:DEL:ALL", "Read Callback"="", "Write Callback"="", "Range Callback"="", "Check Callback"="", "Rngtable Callback"="", "Coerce Callback"="", "User Callback"="", "Supported Models"="", "Instrument Options"="", "Repeated Capabilities"="", "Restricted Repeated Capabilities"="", "Help"="This attribute deletes all sweep segments in the channel (Del. All Segments).\n\nAvailable Repeated Capabilities:\nChannel: CH1,CH2,CH3,CH4,CH5,CH6,CH7,CH8,CH9,CH10,CH11,CH12,CH13,CH14,CH15,CH16,CH17,CH18,CH19,CH20\r\n\nRemote-control command(s):\n[SENSe<Ch>:]SEGMent:DELete:ALL", "Flags"={"OPC Wait"=FALSE, "Dont check status"=FALSE, "*WAI"=FALSE}, "Check Status Callback"=""}, {"Level"=3, "Descriptive Name"="NWA Segment Get Frequency Center", "Class Only"=FALSE, "Data Type"=1, "Access"=0, "Identifier"="RSZVL_ATTR_NWA_SEGMENT_GET_FREQ_CENTER", "Range Table"="", "Command"="SENS{Channel}:SEGM{Segment}:FREQ:CENT?", "Read Callback"="", "Write Callback"="", "Range Callback"="", "Check Callback"="", "Rngtable Callback"="", "Coerce Callback"="", "User Callback"="", "Supported Models"="", "Instrument Options"="", "Repeated Capabilities"="", "Restricted Repeated Capabilities"="", "Help"="This attribute returns the center frequency of sweep segment no. <Seg>.\n\nAvailable Repeated Capabilities:\nChannel: CH1,CH2,CH3,CH4,CH5,CH6,CH7,CH8,CH9,CH10,CH11,CH12,CH13,CH14,CH15,CH16,CH17,
